vi "TEST Multiple Errors Exp1.vi"() -> ()   [LabVIEW 2020, in "Multiple Errors.lvclass"]
uses:
  Multiple Errors.lvclass
  <vilib>/Utility/error.llb/Error Cluster From Error Code.vi
  <vilib>/ErrorRing/Error Ring.xnode
  <vilib>/MultiError/TokenizeJSON/Multi Error Cluster.lvlib
panel:
  out "error out 2":errorcluster
  out "error out":errorcluster
  out "attribute names":string[](array[string])
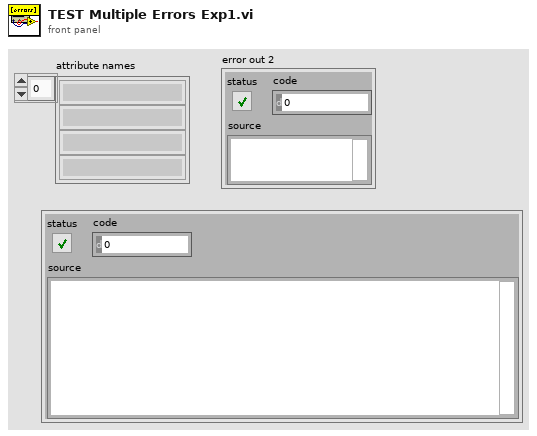
[diagram p1: front panel]
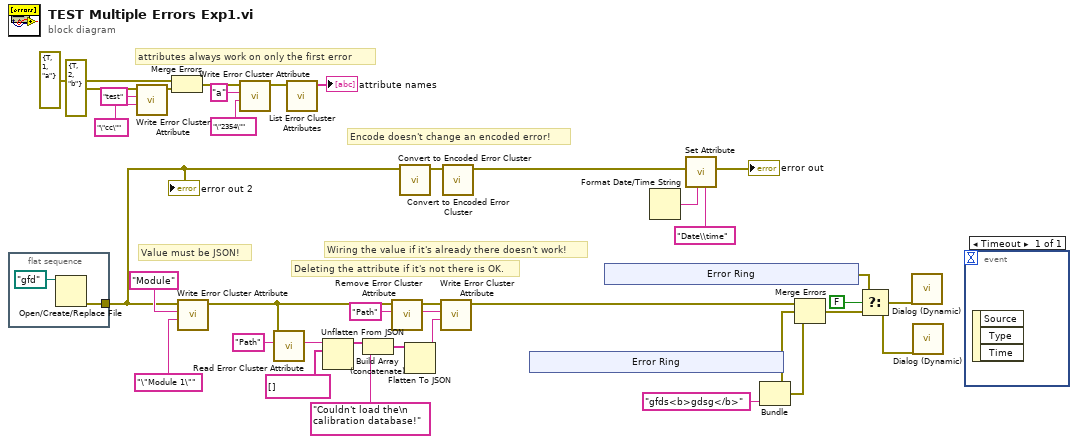
[diagram p0: block diagram]
diagram:
  w18 = "Path" ("attribute name")
  # "attributes always work on only the first error"
  # "Encode doesn't change an encoded error!"
  # "Deleting the attribute if it's not there is OK."
  # "Wiring the value if it's already there doesn't work!"
  # "Value must be JSON!"
  n1 = flat-sequence {
    tunnel: [w38] -> w14
    frame #0 {
      n2 = Open/Create/Replace File(file path (use dialog)=path "gfd") -> (error out=w38:errorcluster)  [unwired: 5 in, 2 out]
    }
  }
  n3 = call <vilib>:"Write Error Cluster Attribute.vi"("JSON value"="\"cc\"" ("attribute name"), "attribute name"="test", "error in"=errorcluster {"status"=TRUE, "code"=2, "source"="b"}) -> ("error out"=w30:errorcluster)  [unwired: 7 in, 1 out]
  n4 = Merge Errors(errorcluster {"status"=TRUE, "code"=1, "source"="a"} ("error in"), w30) -> (w29:errorcluster)
  n5 = call <vilib>:"Write Error Cluster Attribute.vi"("JSON value"="\"Module 1\"" ("attribute name"), "attribute name"="Module", "error in"=w14) -> ("error out"=w17:errorcluster)  [unwired: 7 in, 1 out]
  n6 = call <vilib>:"Write Error Cluster Attribute.vi"("JSON value"="\"2354\"" ("attribute name"), "attribute name"="a", "error in"=w29) -> ("error out"=w27:errorcluster)  [unwired: 7 in, 1 out]
  n7 = call <vilib>:"Read Error Cluster Attribute.vi"("attribute name"="Path", "error"=w17) -> ("value string"=w24:string)  [unwired: 7 in, 2 out]
  n8 = call <vilib>:"List Error Cluster Attributes.vi"("error"=w27) -> ("attribute names"=→"attribute names":string[])  [unwired: 10 in]
  n9 = Unflatten From JSON(JSON string=w24, type and defaults=string[] []) -> (value=w22:string[])  [unwired: 5 in, 1 out]
  n10 = Build Array (concatenate)(w22, "Couldn't load the\n calibration database!" ("attribute name")) -> (w20:string[])
  n11 = call <vilib>:"Remove Error Cluster Attribute.vi"("attribute name"=w18, "error in"=w17) -> ("error out"=w16:errorcluster)  [unwired: 8 in, 1 out]
  n12 = call <vilib>:"Convert to Encoded Error Cluster.vi"("error in"=w14) -> ("error out"=w13:errorcluster)  [unwired: 10 in]
  n13 = Flatten To JSON(anything=w20) -> (JSON string=w19:string)  [unwired: 2 in, 1 out]
  n14 = call <vilib>:"Write Error Cluster Attribute.vi"("JSON value"=w19, "attribute name"=w18, "error in"=w16) -> ("error out"=w15:errorcluster)  [unwired: 7 in, 1 out]
  n15 = call <vilib>:"Convert to Encoded Error Cluster.vi"("error in"=w13) -> ("error out"=w3:errorcluster)  [unwired: 10 in]
  n16 = xnode "Error Ring"() -> ("error out"=w10:errorcluster)
  n17 = xnode "Error Ring"() -> ("error out"=w7:errorcluster)
  n18 = Format Date/Time String() -> (date/time string=w4:string)  [unwired: 3 in]
  n19 = call "Set Attribute.vi"("Attribute [\"Info\"]"="Date\\time" ("Attribute [\"Info\"]"), "Text"=w4, "error in (no error)"=w3) -> ("error out"=→"error out":errorcluster)  [unwired: 8 in]
  n20 = Bundle(cluster=w10, "source"="gfds<b>gdsg</b>") -> (w9:errorcluster)  [unwired: 2 in]
  n21 = Merge Errors(w15, w10, w9) -> (w8:errorcluster)
  n22 = Select(t=w7, s=FALSE, f=w8) -> (s? t:f=w1:errorcluster)
  n23 = call "Dialog (Dynamic).vi"("error in (no error)"=w1) -> ()  [unwired: 10 in, 1 out]
  n24 = call "Dialog (Dynamic).vi"("error in (no error)"=w1) -> ()  [unwired: 10 in, 1 out]
  n25 = event shown="[0] Timeout" {
    selector: _ -> [_]
    dyn-events: _ -> [_]
    timeout: _ -> [_]
    event Timeout {
      n26 = event-data() -> ()  [unwired: 1 in, 3 out]
    }
  }
  "error out 2" <- w14
